vi "matchPatternCaseInsensitive.vi"(10 "String":string, 11 "Command 4":string) -> (2 "match":string, 3 "after":string, 5 "before":string)   [LabVIEW 2011]
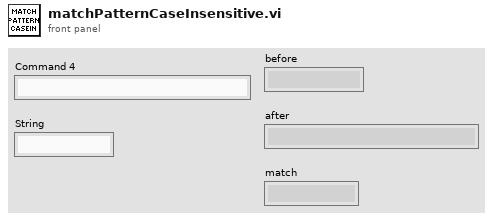
[diagram p1: front panel]
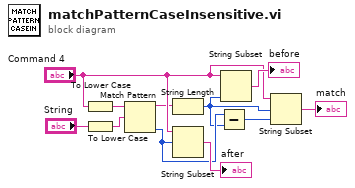
[diagram p0: block diagram]
diagram:
  n1 = To Lower Case(string="Command 4") -> (all lower case string=w4:string)
  n2 = To Lower Case(string="String") -> (all lower case string=w3:string)
  n3 = Match Pattern(string=w4, regular expression=w3) -> (before substring=w1:string, offset past match=w7:i32)  [unwired: 1 in, 2 out]
  n4 = String Length(string=w1) -> (length=w5:i32)
  n5 = String Subset(string="Command 4", offset (0)=w7) -> (substring=→"after":string)  [unwired: 1 in]
  n6 = Subtract(x=w7, y=w5) -> (x-y=w6:i32)
  n7 = String Subset(string="Command 4", length (rest)=w5) -> (substring=→"before":string)  [unwired: 1 in]
  n8 = String Subset(string="Command 4", offset (0)=w5, length (rest)=w6) -> (substring=→"match":string)
